vi "Run.vi"(8 "error in (no error)":errorcluster, 11 "PmuCalCal in":refnum<class "PmuCalCal.lvclass">) -> (0 "error out":errorcluster, 1 "DataValid":bool, 2 "clSensorData":T1, 3 "PmuCalCal out":refnum<class "PmuCalCal.lvclass">)   [LabVIEW 2018, in "SensorPlugins.lvlib" / "PmuCalCal.lvclass"]
uses:
  PmuCalCal.lvclass
  C:/Users/ico/Documents/Projects/NistPluggableModules/Sensor/SensorPlugins/PmuBaseClass/PmuBase.lvclass
  SensorShared/clSensorData.ctl
  PmuBaseClass/Typedef/PmuData.ctl
  PmuBaseClass/PmuBase.lvclass/PmuBase.ctl
  PmuBaseClass/Accessors/Read PmuConfig.vi
  PmuBaseClass/Accessors/Write PmuConfig.vi
  SensorShared/SensorShared.lvlib
  PmuBaseClass/PmuBase.lvclass
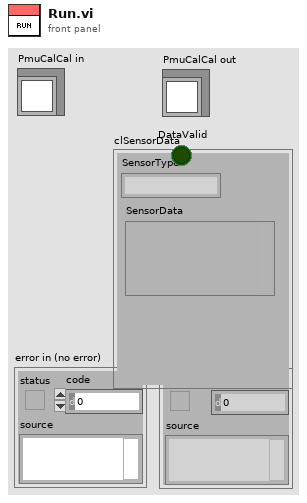
[diagram p1: front panel]
types:
  T1 = typedef "SensorShared.lvlib/clSensorData.ctl" = cluster{"SensorType":string, "SensorData":variant}
  T2 = typedef "SensorPlugins.lvlib/PmuBase.lvclass/PmuData.ctl" = cluster{"Timestamp":dbl, "Synx":cdb[], "Freq":dbl, "ROCOF":dbl, "ID":i16}
  T3 = typedef "SensorPlugins.lvlib/PmuBase.lvclass/PmuConfig.ctl" = cluster{"Class":enum16{"M", "P"}, "Fs":i32, "F0":i32, "FSamp":i32, "SettlingTime":dbl, "T0":ext}
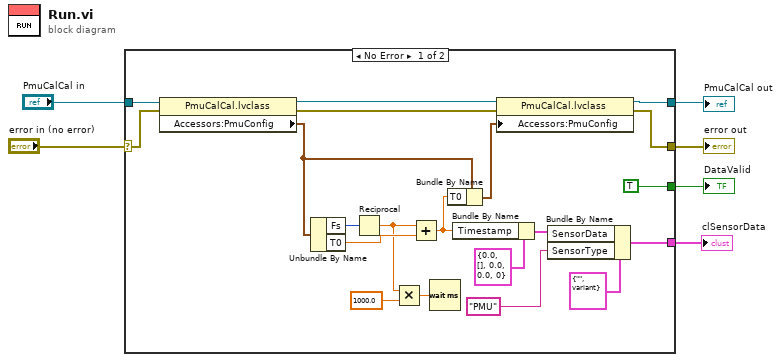
[diagram p0: block diagram]
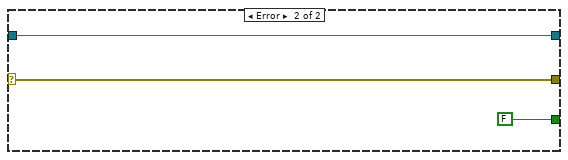
[diagram p2: hidden frame]
diagram:
  n1 = case shown="No Error" "error in (no error)" {
    selector: "error in (no error)" -> [w25 w29]
    tunnel: [w7 w29] -> w5
    tunnel: [w12 w28] -> w3
    tunnel: "PmuCalCal in" -> [w26 w28]
    tunnel: [TRUE ("DataValid") FALSE ("DataValid")] -> w2
    tunnel: [w13 _] -> w1
    frame No Error {
      n2 = property class="PmuCalCal.lvclass"(reference=w26, error in=w25) -> (reference out=w11:refnum<class "PmuCalCal.lvclass">, error out=w10:errorcluster, "Accessors:PmuConfig"=w22:T3)
      n3 = Unbundle By Name(w22) -> ("Fs"=w24:i32, "T0"=w23:ext)
      n4 = Reciprocal(x=w24) -> (1/x=w14:dbl)
      n5 = Multiply(x=w14, y=1000.0) -> (x*y=w16:dbl)
      n6 = Add(x=w14, y=w23) -> (x+y=w19:ext)
      n7 = Wait (ms)(milliseconds to wait=w16) -> ()  [unwired: 1 out]
      n8 = Bundle By Name(cluster=w22, "T0"=w19) -> (w9:T3)
      n9 = Bundle By Name(cluster=T2 {"Timestamp"=0.0, "Synx"=[], "Freq"=0.0, "ROCOF"=0.0, "ID"=0} ("PmuReport"), "Timestamp"=w19) -> (w17:T2)
      n10 = property class="PmuCalCal.lvclass"(reference=w11, error in=w10, "Accessors:PmuConfig"=w9) -> (reference out=w12:refnum<class "PmuCalCal.lvclass">, error out=w7:errorcluster)
      n11 = Bundle By Name(cluster=T1 {"SensorType"="", "SensorData"=variant} ("clSensorData"), "SensorData"=w17, "SensorType"="PMU") -> (w13:T1)
    }
    frame Error {
    }
  }
  "error out" <- w5
  "PmuCalCal out" <- w3
  "clSensorData" <- w1
  "DataValid" <- w2
